vi "Get Test Mode.vi"(8 "error in (no error)":errorcluster, 11 "NF in":refnum<class "NF.lvclass">) -> (0 "error out":errorcluster, 2 "Test Mode":string, 3 "NF out":refnum<class "NF.lvclass">)   [LabVIEW 2018, in "NF.lvlib" / "NF.lvclass"]
uses:
  NF.lvclass
  C:/Sequence Automation/Plugins/Measurement Interface.lvlibp/Measurement Interface.lvclass
  Plugins/Measurement Interface.lvlibp/Private Methods/Measurement Parameters/Read Measurement Parameters.vi
  Plugins/String Database.lvlibp/String Database.lvclass
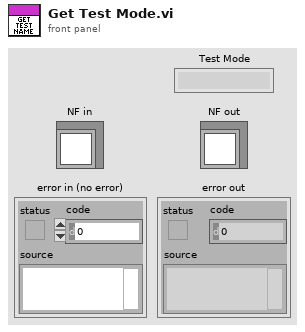
[diagram p1: front panel]
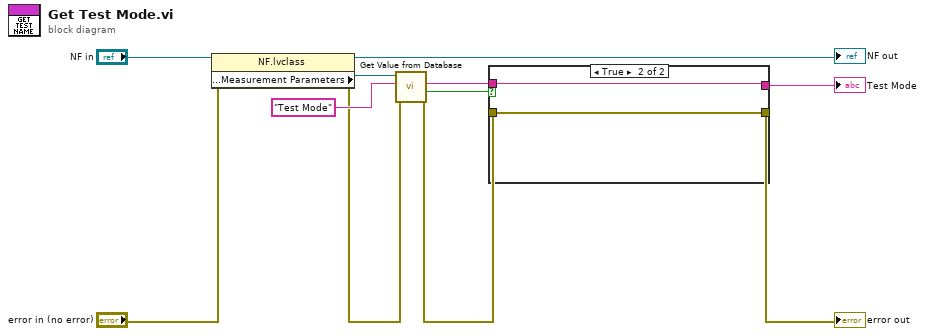
[diagram p0: block diagram]
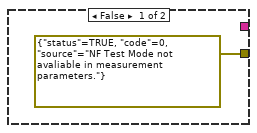
[diagram p2: hidden frame]
diagram:
  n1 = property class="NF.lvclass"(reference="NF in", error in="error in (no error)") -> (reference out=→"NF out":refnum<class "NF.lvclass">, error out=w9:errorcluster, "Protected Methods:Measurement Parameters"=w11:refnum<class "String Database.lvclass">)
  n2 = call "Get Value from Database.vi"("error in (no error)"=w9, "Entry Name"="Test Mode", "Message in"=w11) -> ("error out"=w7:errorcluster, "Entry Found"=w8:bool, "Entry Value"=w6:string)  [unwired: 5 in, 1 out]
  n3 = case shown="True" w8 {
    tunnel: w7 -> [_ w13]
    tunnel: [errorcluster {"status"=TRUE, "code"=0, "source"="NF Test Mode not avaliable in measurement parameters."} ("error out") w13] -> w2
    tunnel: w6 -> [_ w14]
    tunnel: [_ w14] -> w1
    frame False {
    }
    frame True {
    }
  }
  "error out" <- w2
  "Test Mode" <- w1
